vi "Write Events.vi"(8 "error in (no error)":errorcluster, 10 "Events":T1, 11 "DAQ Data in":refnum<class "DAQ Data.lvclass">) -> (0 "error out":errorcluster, 3 "DAQ Data out":refnum<class "DAQ Data.lvclass">)   [LabVIEW 2022 SP3, in "DAQ Data.lvclass"]
uses:
  DAQ Data.lvclass
  DAQ Data.lvclass/DAQ Data.ctl
  AIDAQ Data.ctl
  AI Daq Data.lvlib
  Events.ctl
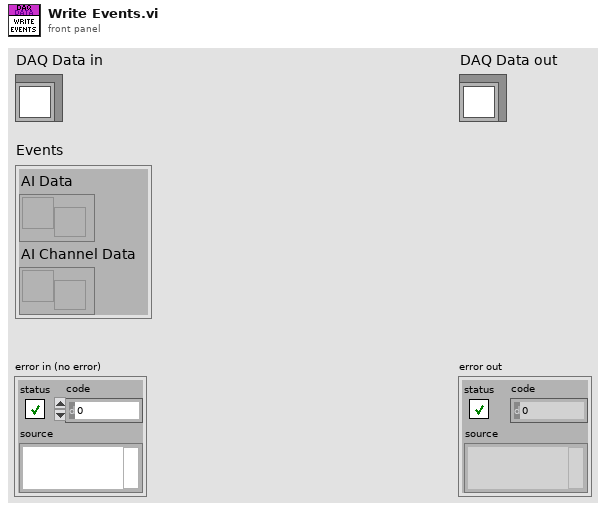
[diagram p1: front panel]
types:
  T1 = typedef "DAQ Data.lvclass/Events.ctl" = cluster{"AI Data":refnum<user-event>, "AI Channel Data":refnum<user-event>}
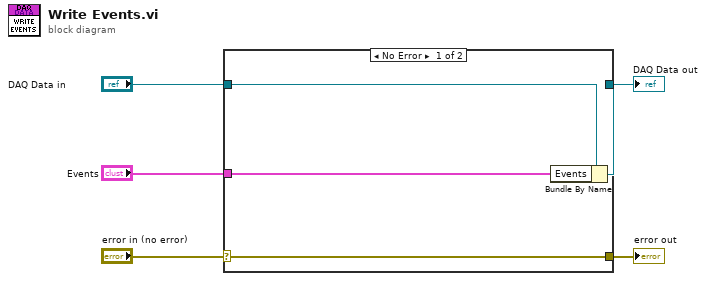
[diagram p0: block diagram]
diagram:
  n1 = case shown="No Error" "error in (no error)" {
    selector: "error in (no error)" -> [w9 w10]
    tunnel: [w9 w10] -> w4
    tunnel: [w7 w11] -> w2
    tunnel: "DAQ Data in" -> [w8 w11]
    tunnel: "Events" -> [w6 _]
    frame No Error {
      n2 = Bundle By Name(cluster=w8, "Events"=w6) -> (w7:refnum<class "DAQ Data.lvclass">)
    }
    frame Error {
    }
  }
  "error out" <- w4
  "DAQ Data out" <- w2
